vi "Manual Mode(not too old).vi"(5 "Shooter":dbl, 6 "Climb?":bool, 7 "Shooter":T1, 8 "engage shoot":bool, 9 "Potent":dbl, 11 "Button 1":bool) -> ()   [LabVIEW 2012]
uses:
  <vilib>/Rock Robotics/WPI/Solenoid/WPI_SolenoidValue.ctl
  <vilib>/Rock Robotics/WPI/RobotDrive/WPI_RobotDriveArcadeDrive_Standard(NoSaturation).vi
  <vilib>/Rock Robotics/WPI/RobotDrive/WPI_RobotDriveGetSetRefNum.vi
  <vilib>/Rock Robotics/WPI/Solenoid/WPI_SolenoidSetEnum.vi
  <vilib>/Rock Robotics/WPI/Joystick/WPI_JoystickGetSetRefNum.vi
panel:
  in  "Shooting Pitch":dbl
  out "Red":dbl[](array[numeric])
  out "Green":dbl[](array[numeric])
  out "Yellow":dbl[](array[numeric])
  in  "Kick?":bool
  out "green":dbl
  out "yellow":dbl
  out "red":dbl
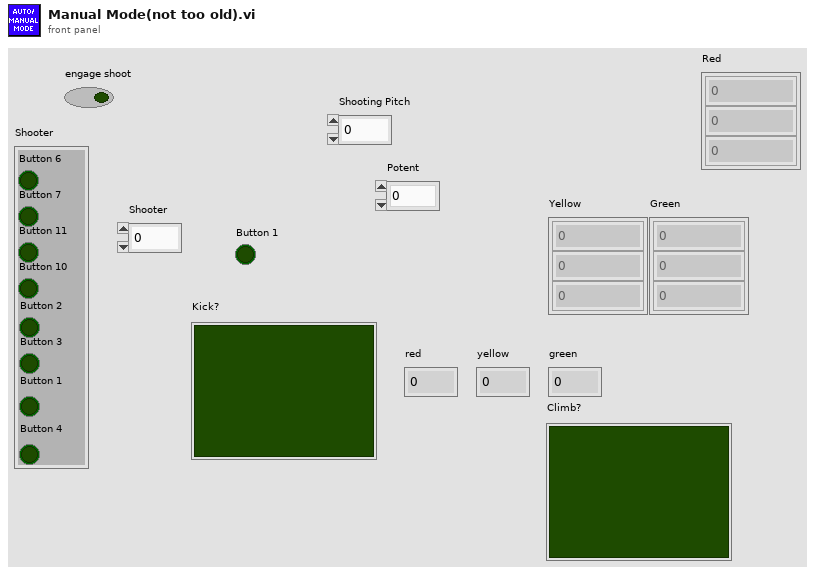
[diagram p1: front panel]
types:
  T1 = cluster{"Button 6":bool, "Button 7":bool, "Button 11":bool, "Button 10":bool, "Button 2":bool, "Button 3":bool, "Button 1":bool, "Button 4":bool}
  T2 = typedef "WPI_SolenoidDevRef.ctl" = cluster{"DevStatus":errorcluster, "Solenoid Module":T3, "Forward Solenoid Channel":T4, "Reverse Solenoid Channel":T4}
  T3 = typedef "FPGA_TypedefSolenoidModule.ctl" = enum16{"Solenoid Module 1", "Solenoid Module 2"}
  T4 = typedef "WPI_SolenoidChannel.ctl" = enum8{"Solenoid 1", "Solenoid 2", "Solenoid 3", "Solenoid 4", "Solenoid 5", "Solenoid 6", "Solenoid 7", "Solenoid 8", "Invalid"}
  T5 = typedef "WPI_JoystickDevRef.ctl" = cluster{"Device":T6}
  T6 = typedef "WPI_JoystickDeviceEnum.ctl" = enum16{"USB 1", "USB 2", "USB 3", "USB 4", "Kinect 1", "Kinect 2"}
  T7 = typedef "WPI_JoystickButtonState.ctl" = cluster{"Button 1":bool, "Button 2":bool, "Button 3":bool, "Button 4":bool, "Button 5":bool, "Button 6":bool, "Button 7":bool, "Button 8":bool, "Button 9":bool, "Button 10":bool, "Button 11":bool, "Button 12":bool}
  T8 = typedef "WPI_MotorControlDeviceRef.ctl" = cluster{"DeviceStatus":errorcluster, "Type":enum16{"PWM", "CAN"}, "PWM":cluster{"Digital Module":T9, "PWM Channel":T10, "DeadBand":T11}, "CAN":cluster{"Device Number":u8, "Control Mode":T12, "Semaphore":T13, "Max Vout":dbl}, "Invert":bool, "TransformRef":T14, "InvTransformRef":T14}
  T9 = typedef "FPGA_TypedefDigitalModule.ctl" = enum16{"Digital Module 1", "Digital Module 2"}
  T10 = typedef "FPGA_DIOPWMChannel.ctl" = enum8{"PWM 1", "PWM 2", "PWM 3", "PWM 4", "PWM 5", "PWM 6", "PWM 7", "PWM 8", "PWM 9", "PWM 10", "Invalid"}
  T11 = typedef "WPI_PWMDeadband.ctl" = cluster{"Name":string, "maxPositivePwm":i32, "minPositivePwm":i32, "centerPwm":i32, "maxNegativePwm":i32, "minNegativePwm":i32, "angularRange":u16}
  T12 = typedef "WPI_CANJaguar_ControlMode.ctl" = enum8{"Percent VBus", "Current", "Speed", "Position", "Voltage"}
  T13 = typedef "Semaphore RefNum" = refnum<k1>
  T14 = typedef "WPI_PWMTransform_ConPane.ctl" = refnum<vi>
  T15 = typedef "WPI_SolenoidValue.ctl" = enum16{"Off", "On", "Forward", "Reverse"}
  T16 = typedef "WPI_RobotDriveDevRef.ctl" = cluster{"DevStatus":errorcluster, "Motors[]":T8[], "Square Inputs":bool, "Max Output":dbl, "Isochronous":bool}
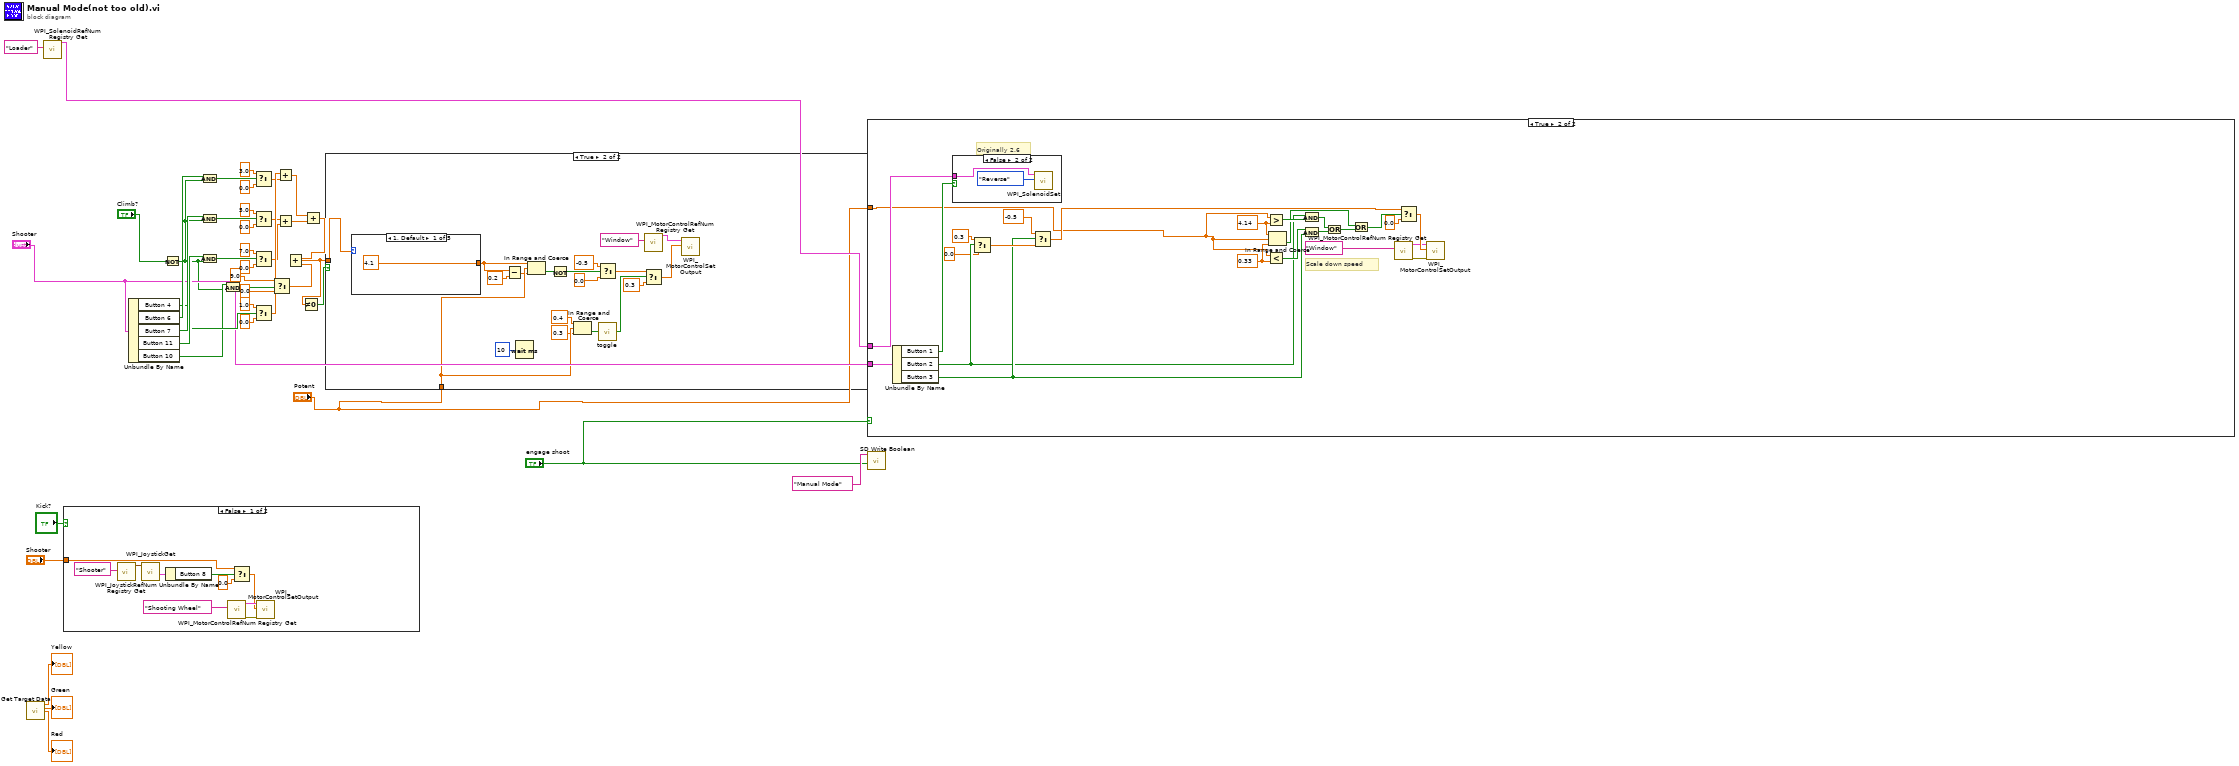
[diagram p0: block diagram]
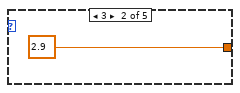
[diagram p3: hidden frame]
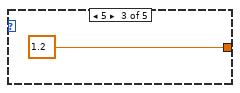
[diagram p4: hidden frame]
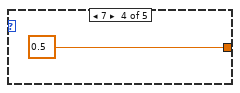
[diagram p5: hidden frame]
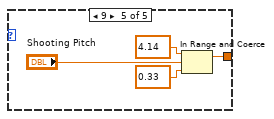
[diagram p6: hidden frame]
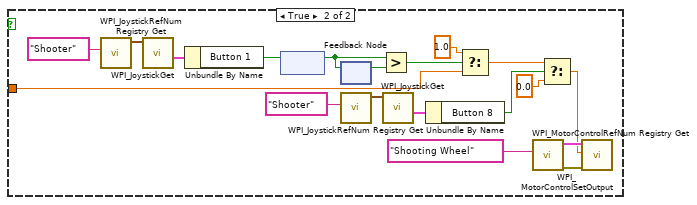
[diagram p7: hidden frame]
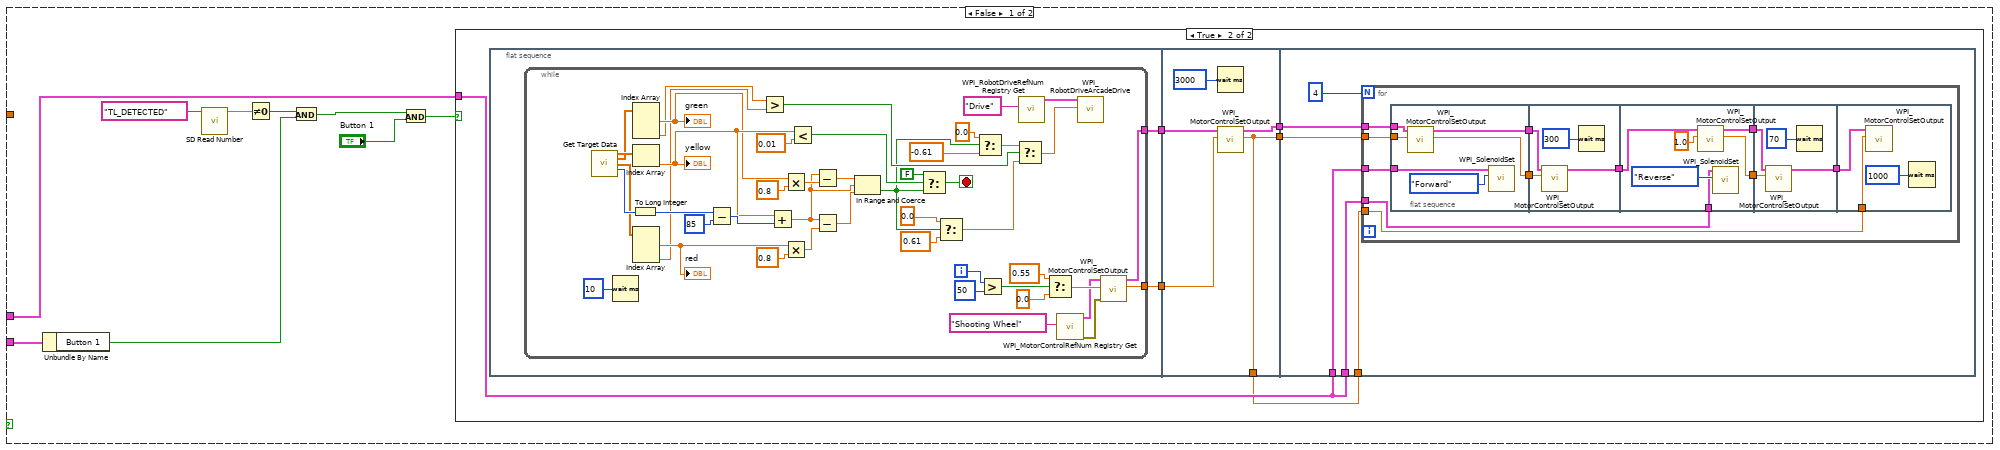
[diagram p8: hidden frame]
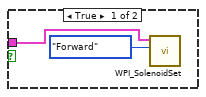
[diagram p10: hidden frame]
diagram:
  n1 = call "Get Target Data.vi"() -> ("Yellow"=→"Yellow":dbl[], "Green"=→"Green":dbl[], "Red"=→"Red":dbl[])  [unwired: 11 in, 2 out]
  n2 = call <vilib>:"WPI_SolenoidRefNum Registry Get.vi"("refnum name"="Loader") -> ("SolenoidDevRef"=w41:T2)  [unwired: 9 in, 1 out]
  n3 = case shown="False" "Kick?" {
    tunnel: "Shooter" -> [w43 w53]
    frame False {
      n4 = call <vilib>:"WPI_JoystickRefNum Registry Get.vi"("refnum name"="Shooter") -> ("JoystickDevRef"=w49:T5)  [unwired: 9 in, 1 out]
      n5 = call <vilib>:"WPI_JoystickGet.vi"("JoystickDevRef"=w49) -> ("Buttons"=w50:T7)  [unwired: 4 in, 2 out]
      n6 = Unbundle By Name(w50) -> ("Button 8"=w44:bool)
      n7 = call <vilib>:"WPI_MotorControlRefNum Registry Get.vi"("refnum name"="Shooting Wheel") -> ("error out"=w52:errorcluster, "MotorControlDevRef"=w47:T8)  [unwired: 9 in]
      n8 = Select(t=w43, s=w44, f=0.0) -> (s? t:f=w46:dbl)
      n9 = call <vilib>:"WPI_MotorControlSetOutput.vi"("error in (no error)"=w52, "Output"=w46, "MotorControlDevRef"=w47) -> ()  [unwired: 6 in, 3 out]
    }
    frame True {
      n10 = call <vilib>:"WPI_JoystickRefNum Registry Get.vi"("refnum name"="Shooter") -> ("JoystickDevRef"=w71:T5)  [unwired: 9 in, 1 out]
      n11 = call <vilib>:"WPI_JoystickGet.vi"("JoystickDevRef"=w71) -> ("Buttons"=w54:T7)  [unwired: 4 in, 2 out]
      n12 = Unbundle By Name(w54) -> ("Button 1"=w58:bool)
      n13 = feedback #1() -> (w56:bool)  [unwired: 1 in]
      n14 = feedback-in #1(w58) -> ()
      n15 = feedback #2() -> (w55:bool)  [unwired: 1 in]
      n16 = feedback-in #2(w56) -> ()
      n17 = call <vilib>:"WPI_JoystickRefNum Registry Get.vi"("refnum name"="Shooter") -> ("JoystickDevRef"=w66:T5)  [unwired: 9 in, 1 out]
      n18 = Greater?(x=w56, y=w55) -> (0:w57:bool)
      n19 = call <vilib>:"WPI_JoystickGet.vi"("JoystickDevRef"=w66) -> ("Buttons"=w67:T7)  [unwired: 4 in, 2 out]
      n20 = Unbundle By Name(w67) -> ("Button 8"=w61:bool)
      n21 = Select(t=1.0, s=w57, f=w53) -> (s? t:f=w60:dbl)
      n22 = call <vilib>:"WPI_MotorControlRefNum Registry Get.vi"("refnum name"="Shooting Wheel") -> ("error out"=w69:errorcluster, "MotorControlDevRef"=w64:T8)  [unwired: 9 in]
      n23 = Select(t=w60, s=w61, f=0.0) -> (s? t:f=w63:dbl)
      n24 = call <vilib>:"WPI_MotorControlSetOutput.vi"("error in (no error)"=w69, "Output"=w63, "MotorControlDevRef"=w64) -> ()  [unwired: 6 in, 3 out]
    }
  }
  n25 = Unbundle By Name("Shooter") -> ("Button 4"=w13:bool, "Button 6"=w15:bool, "Button 7"=w14:bool, "Button 11"=w33:bool, "Button 10"=w11:bool)
  n26 = Not(x="Climb?") -> (.not. x?=w10:bool)
  n27 = And(x=w15, y=w10) -> (x .and. y?=w32:bool)
  n28 = And(x=w14, y=w10) -> (x .and. y?=w31:bool)
  n29 = And(x=w33, y=w10) -> (x .and. y?=w30:bool)
  n30 = And(x=w11, y=w10) -> (x .and. y?=w7:bool)
  n31 = Select(t=3.0, s=w32, f=0.0) -> (s? t:f=w24:dbl)
  n32 = Select(t=5.0, s=w31, f=0.0) -> (s? t:f=w23:dbl)
  n33 = Select(t=7.0, s=w30, f=0.0) -> (s? t:f=w22:dbl)
  n34 = Select(t=1.0, s=w13, f=0.0) -> (s? t:f=w25:dbl)
  n35 = Select(t=9.0, s=w7, f=0.0) -> (s? t:f=w5:dbl)
  n36 = Add(x=w25, y=w24) -> (x+y=w21:dbl)
  n37 = Add(x=w23, y=w22) -> (x+y=w20:dbl)
  n38 = Add(x=w21, y=w20) -> (x+y=w6:dbl)
  n39 = Add(x=w6, y=w5) -> (x+y=w2:dbl)
  n40 = Not Equal To 0?(x=w2) -> (x != 0?=w1:bool)
  n41 = case shown="True" w1 {
    tunnel: w2 -> [_ w90]
    tunnel: "Potent" -> [_ w89]
    frame False {
    }
    frame True {
      n42 = case shown="1, Default" w90 {
        tunnel: [4.1 ("t") 2.9 ("t") 1.2 ("t") 0.5 ("t") w95] -> w77
        frame 1, Default {
        }
        frame 3 {
        }
        frame 5 {
        }
        frame 7 {
        }
        frame 9 {
          n43 = In Range and Coerce(upper limit=4.14, x="Shooting Pitch", lower limit=0.33) -> (coerced(x)=w95:dbl)  [unwired: 1 out]
        }
      }
      n44 = Subtract(x=w77, y=0.2) -> (x-y=w76:dbl)
      n45 = Wait (ms)(milliseconds to wait=u32 10) -> ()  [unwired: 1 out]
      n46 = In Range and Coerce(upper limit=w77, x=w89, lower limit=w76) -> (In Range?=w75:bool)  [unwired: 1 out]
      n47 = Not(x=w75) -> (.not. x?=w74:bool)
      n48 = In Range and Coerce(upper limit=0.4, x=w89, lower limit=0.3) -> (In Range?=w80:bool)  [unwired: 1 out]
      n49 = call "toggle.vi"("Btn In"=w80) -> ("Toggle Out"=w79:bool)
      n50 = Select(t=-0.5, s=w74, f=0.0) -> (s? t:f=w81:dbl)
      n51 = Select(t=w81, s=w79, f=0.3) -> (s? t:f=w83:dbl)
      n52 = call <vilib>:"WPI_MotorControlRefNum Registry Get.vi"("refnum name"="Window") -> ("MotorControlDevRef"=w87:T8)  [unwired: 9 in, 1 out]
      n53 = call <vilib>:"WPI_MotorControlSetOutput.vi"("Output"=w83, "MotorControlDevRef"=w87) -> ()  [unwired: 7 in, 3 out]
    }
  }
  n54 = case shown="True" "engage shoot" {
    tunnel: "Shooter" -> [w107 w213]
    tunnel: w41 -> [w104 w214]
    tunnel: "Potent" -> [_ w208]
    frame False {
      n55 = Unbundle By Name(w107) -> ("Button 1"=w103:bool)
      n56 = call <vilib>:"SD Read Number.vi"("Name"="TL_DETECTED") -> ("Numeric"=w99:dbl)  [unwired: 8 in, 2 out]
      n57 = Not Equal To 0?(x=w99) -> (x != 0?=w100:bool)
      n58 = And(x=w100, y=w103) -> (x .and. y?=w102:bool)
      n59 = And(x=w102, y="Button 1") -> (x .and. y?=w106:bool)
      n60 = case shown="True" w106 {
        tunnel: w104 -> [_ w113]
        frame False {
        }
        frame True {
          n61 = flat-sequence {
            tunnel: [w115] -> w109
            tunnel: [w114] -> w108
            tunnel: [w164] -> w112
            tunnel: [w165] -> w111
            tunnel: [w164] -> w110
            tunnel: w109 -> [w163]
            tunnel: w108 -> [w162]
            tunnel: w113 -> [w172]
            tunnel: w113 -> [w171]
            tunnel: w112 -> [w169]
            tunnel: w111 -> [w168]
            tunnel: w110 -> [w167]
            frame #0 {
              n62 = while {
                tunnel: [w128] -> w115
                tunnel: [w116] -> w114
                i -> [w134]
                stop <- w150 stop-if-true
                n63 = call "Get Target Data.vi"() -> ("Yellow"=w149:dbl[], "Green"=w147:dbl[], "Red"=w146:dbl[], "x angle"=w148:u16)  [unwired: 11 in, 1 out]
                n64 = Wait (ms)(milliseconds to wait=u32 10) -> ()  [unwired: 1 out]
                n65 = To Long Integer(number=w148) -> (32bit integer=w157:i32)
                n66 = Index Array(array=w147) -> (element #1=w141:dbl, element #3=w126:dbl)  [unwired: 3 in, 1 out]
                "green" <- w141
                n67 = Index Array(array=w149) -> (element=w154:dbl)  [unwired: 1 in]
                "yellow" <- w154
                n68 = Index Array(array=w146) -> (element #1=w143:dbl, element #3=w125:dbl)  [unwired: 3 in, 1 out]
                "red" <- w143
                n69 = Subtract(x=w157, y=85) -> (x-y=w155:i32)
                n70 = Greater?(x=w126, y=w125) -> (0:w124:bool)
                n71 = Add(x=w154, y=w155) -> (x+y=w127:dbl)
                n72 = Multiply(x=w141, y=0.8) -> (x*y=w139:dbl)
                n73 = Multiply(x=w143, y=0.8) -> (x*y=w138:dbl)
                n74 = Less?(x=w154, y=0.01) -> (x < y?=w152:bool)
                n75 = Subtract(x=w127, y=w139) -> (x-y=w144:dbl)
                n76 = Subtract(x=w127, y=w138) -> (x-y=w145:dbl)
                n77 = In Range and Coerce(upper limit=w144, x=w127, lower limit=w145) -> (In Range?=w118:bool)  [unwired: 1 out]
                n78 = Select(t=FALSE, s=w152, f=w118) -> (s? t:f=w150:bool)
                n79 = Select(t=0.0, s=w118, f=0.61) -> (s? t:f=w117:dbl)
                n80 = Select(t=0.0, s=w118, f=-0.61) -> (s? t:f=w121:dbl)
                n81 = Greater?(x=w134, y=50) -> (0:w132:bool)
                n82 = Select(t=w121, s=w124, f=w117) -> (s? t:f=w158:dbl)
                n83 = call <vilib>:"WPI_RobotDriveRefNum Registry Get.vi"("refnum name"="Drive") -> ("RobotDriveDevRef"=w160:T16)  [unwired: 9 in, 1 out]
                n84 = Select(t=0.55, s=w132, f=0.0) -> (s? t:f=w135:dbl)
                n85 = call <vilib>:"WPI_MotorControlRefNum Registry Get.vi"("refnum name"="Shooting Wheel") -> ("error out"=w137:errorcluster, "MotorControlDevRef"=w129:T8)  [unwired: 9 in]
                n86 = call-poly <vilib>:"WPI_RobotDriveArcadeDrive.vi"("X axis value"=w158, "RobotDriveDevRef"=w160) -> ()  [unwired: 7 in, 3 out]
                n87 = call <vilib>:"WPI_MotorControlSetOutput.vi"("error in (no error)"=w137, "Output"=w135, "MotorControlDevRef"=w129) -> ("Motor Output"=w116:dbl, "MotorControlDevRef"=w128:T8)  [unwired: 6 in, 1 out]
              }
            }
            frame #1 {
              n88 = Wait (ms)(milliseconds to wait=u32 3000) -> ()  [unwired: 1 out]
              n89 = call <vilib>:"WPI_MotorControlSetOutput.vi"("Output"=w162, "MotorControlDevRef"=w163) -> ("Motor Output"=w164:dbl, "MotorControlDevRef"=w165:T8)  [unwired: 7 in, 1 out]
            }
            frame #2 {
              n90 = for {
                N: 4 -> [_]
                tunnel: w172 -> [w177]
                tunnel: w171 -> [w176]
                tunnel: w169 -> [w175]
                tunnel: w168 -> [w174]
                tunnel: w167 -> [w173]
                n91 = flat-sequence {
                  tunnel: [w188] -> w183
                  tunnel: [w187] -> w181
                  tunnel: w177 -> [w186]
                  tunnel: w175 -> [w185]
                  tunnel: w174 -> [w184]
                  tunnel: w183 -> [w192]
                  tunnel: w181 -> [w191]
                  tunnel: [w190] -> w180
                  tunnel: [w197] -> w182
                  tunnel: w180 -> [w196]
                  tunnel: [w195] -> w179
                  tunnel: w176 -> [w194]
                  tunnel: w182 -> [w202]
                  tunnel: w179 -> [w201]
                  tunnel: [w200] -> w178
                  tunnel: w178 -> [w206]
                  tunnel: w173 -> [w204]
                  frame #0 {
                    n92 = call <vilib>:"WPI_MotorControlSetOutput.vi"("Output"=w185, "MotorControlDevRef"=w184) -> ("Motor Output"=w188:dbl, "MotorControlDevRef"=w187:T8)  [unwired: 7 in, 1 out]
                    n93 = call-poly <vilib>:"WPI_SolenoidSet.vi"("Value"=WPI_SolenoidValue."Forward", "SolenoidDevRef"=w186) -> ()  [unwired: 8 in, 2 out]
                  }
                  frame #1 {
                    n94 = call <vilib>:"WPI_MotorControlSetOutput.vi"("Output"=w192, "MotorControlDevRef"=w191) -> ("MotorControlDevRef"=w190:T8)  [unwired: 7 in, 2 out]
                    n95 = Wait (ms)(milliseconds to wait=u32 300) -> ()  [unwired: 1 out]
                  }
                  frame #2 {
                    n96 = call <vilib>:"WPI_MotorControlSetOutput.vi"("Output"=1.0, "MotorControlDevRef"=w196) -> ("Motor Output"=w197:dbl, "MotorControlDevRef"=w195:T8)  [unwired: 7 in, 1 out]
                    n97 = call-poly <vilib>:"WPI_SolenoidSet.vi"("Value"=WPI_SolenoidValue."Reverse", "SolenoidDevRef"=w194) -> ()  [unwired: 8 in, 2 out]
                  }
                  frame #3 {
                    n98 = call <vilib>:"WPI_MotorControlSetOutput.vi"("Output"=w202, "MotorControlDevRef"=w201) -> ("MotorControlDevRef"=w200:T8)  [unwired: 7 in, 2 out]
                    n99 = Wait (ms)(milliseconds to wait=u32 70) -> ()  [unwired: 1 out]
                  }
                  frame #4 {
                    n100 = call <vilib>:"WPI_MotorControlSetOutput.vi"("Output"=w204, "MotorControlDevRef"=w206) -> ()  [unwired: 7 in, 3 out]
                    n101 = Wait (ms)(milliseconds to wait=u32 1000) -> ()  [unwired: 1 out]
                  }
                }
              }
            }
          }
        }
      }
    }
    frame True {
      w222 = 0.33 ("lower limit")
      w226 = 4.14 ("upper limit")
      # "Originally 2.6"
      # "Scale down speed"
      n102 = Unbundle By Name(w213) -> ("Button 1"=w212:bool, "Button 2"=w215:bool, "Button 3"=w216:bool)
      n103 = case shown="False" w212 {
        tunnel: w214 -> [w232 w234]
        frame True {
          n104 = call-poly <vilib>:"WPI_SolenoidSet.vi"("Value"=WPI_SolenoidValue."Forward", "SolenoidDevRef"=w232) -> ()  [unwired: 8 in, 2 out]
        }
        frame False {
          n105 = call-poly <vilib>:"WPI_SolenoidSet.vi"("Value"=WPI_SolenoidValue."Reverse", "SolenoidDevRef"=w234) -> ()  [unwired: 8 in, 2 out]
        }
      }
      n106 = Select(t=0.3, s=w215, f=0.0) -> (s? t:f=w225:dbl)
      n107 = Select(t=-0.5, s=w216, f=w225) -> (s? t:f=w209:dbl)
      n108 = Greater?(x=w208, y=w226) -> (0:w224:bool)
      n109 = Less?(x=w208, y=w222) -> (x < y?=w221:bool)
      n110 = In Range and Coerce(upper limit=w226, x=w208, lower limit=w222) -> (In Range?=w217:bool)  [unwired: 1 out]
      n111 = And(x=w215, y=w224) -> (x .and. y?=w223:bool)
      n112 = And(x=w221, y=w216) -> (x .and. y?=w218:bool)
      n113 = Or(x=w223, y=w218) -> (x .or. y?=w220:bool)
      n114 = Or(x=w217, y=w220) -> (x .or. y?=w219:bool)
      n115 = call <vilib>:"WPI_MotorControlRefNum Registry Get.vi"("refnum name"="Window") -> ("error out"=w227:errorcluster, "MotorControlDevRef"=w228:T8)  [unwired: 9 in]
      n116 = Select(t=w209, s=w219, f=0.0) -> (s? t:f=w229:dbl)
      n117 = call <vilib>:"WPI_MotorControlSetOutput.vi"("error in (no error)"=w227, "Output"=w229, "MotorControlDevRef"=w228) -> ()  [unwired: 6 in, 3 out]
    }
  }
  n118 = call <vilib>:"SD Write Boolean.vi"("Boolean"="engage shoot", "Name"="Manual Mode") -> ()  [unwired: 8 in, 2 out]
